vi "Call.vi"(6 "Error":errorcluster, 10 "Message":T1 {"MessageMetadata"."AbsoluteTime" format="%<%x %.3X>T"}, 11 "Actor":refnum<class "Actor.lvclass">) -> (2 "Message":T1 {"MessageMetadata"."AbsoluteTime" format="%<%x %.3X>T"}, 3 "Actor":refnum<class "Actor.lvclass">, 4 "Error":errorcluster)   [LabVIEW 2020, in "_Template.lvlib" / "MessageTemplate.lvlib" / "{{Name}}.lvlib"]
uses:
  {{Name}}.lvlib
  jettl/jettl/Actor/Actor.lvclass
  ConcreteMessage/ConcreteMessage.lvclass
  jettl/jettl/jettl.lvlib
  jettl/jettl/Lifetime.ctl
  jettl/jettl/TellOrigin.ctl
  jettl/jettl/MessageMetadata.ctl
  Message.ctl
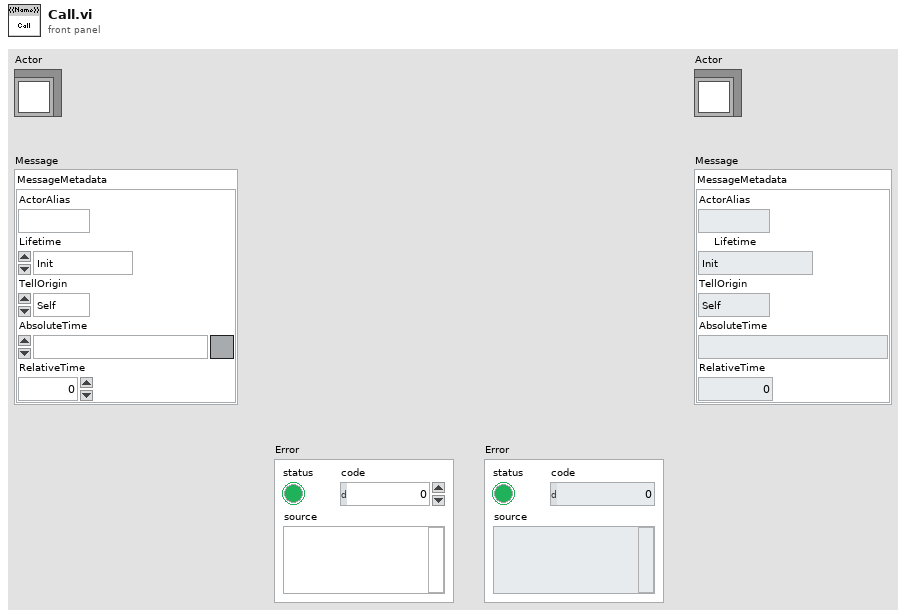
[diagram p1: front panel]
types:
  T1 = typedef "_Template.lvlib/MessageTemplate.lvlib/{{Name}}.lvlib/Message.ctl" = cluster{"MessageMetadata":T2}
  T2 = typedef "jettl.lvlib/MessageMetadata.ctl" = cluster{"ActorAlias":string, "Lifetime":T3, "TellOrigin":T4, "AbsoluteTime":timestamp, "RelativeTime":dbl}
  T3 = typedef "jettl.lvlib/Lifetime.ctl" = enum16{"Init", "Spawn", "Setup", "TeardownBeforeRunning", "Running", "StopCalled", "StoppingWithComponents", "StoppingNoComponents", "TeardownAfterRunning", "Stopped"}
  T4 = typedef "jettl.lvlib/TellOrigin.ctl" = enum16{"Self", "Mediator", "Component"}
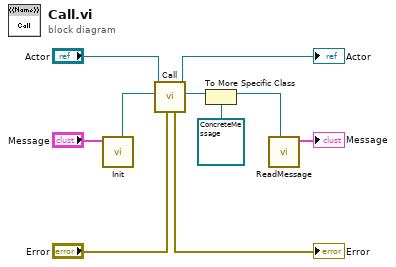
[diagram p0: block diagram]
diagram:
  n1 = call "Init.vi"("Message"="Message") -> ("ConcreteMessage"=w2:refnum<class "ConcreteMessage.lvclass">)  [unwired: 10 in]
  n2 = call "Call.vi"("Error"="Error", "Message"=w2, "Actor"="Actor") -> ("Message"=w4:refnum<class "Message.lvclass">, "Actor"=→"Actor":refnum<class "Actor.lvclass">, "Error"=→"Error":errorcluster)  [unwired: 6 in]
  n3 = To More Specific Class(target class=refnum<class "ConcreteMessage.lvclass"> refnum ("_Template.lvlib:Templates.lvlib:{{Name}}Message.lvlib:{{Name}}Message.lvclass"), reference=w4) -> (specific class reference=w3:refnum<class "ConcreteMessage.lvclass">)  [unwired: 1 in, 1 out]
  n4 = call "ReadMessage.vi"("ConcreteMessage"=w3) -> ("Message"=→"Message":T1)  [unwired: 10 in]
